vi "Double FFT Mesurament (Control - Init Wave&Window - Snapshot - DoubleFFT - Latency - Low Freq) RT Test.vi"() -> ()   [LabVIEW 2014]
uses:
  <vilib>/Platform/TimedLoop/XDataNode/timing_clust.ctl
  <vilib>/Platform/TimedLoop/XDataNode/nitl_modes.ctl
  <vilib>/Platform/TimedLoop/XDataNode/wakeup.ctl
  <vilib>/FPGAPlugInAG/sbRIO-9636/niLvFpga_Open_sbRIO-9636.vi
  <vilib>/rvi/interface/common/dynamic/niFpgaDynamicAddResources.vi
  <vilib>/Utility/error.llb/Error Cluster From Error Code.vi
  <vilib>/rvi/errors/niLvFpgaAdjustHostInterfaceError.vi
  <vilib>/rvi/interface/common/niFpgaWaitOnOcc.vi
  <vilib>/FPGAPlugInAG/Dynamic/niLvFpga_Run_Dynamic.vi
  <vilib>/FPGAPlugInAG/Dynamic/niLvFpga_Abort_Dynamic.vi
  <vilib>/FPGAPlugInAG/Dynamic/niLvFpga_Reset_Dynamic.vi
  <vilib>/FPGAPlugInAG/Dynamic/niLvFpga_Close_Dynamic.vi
  <vilib>/rvi/interface/nirviOpenFPGA/nirviOpenFPGA.xnode
  FPGA Bitfiles/LaserDistanceSen_FPGATarget_DoubleFFTMesuram_744PzgZsl5A.lvbitx
  FPGA Target/Test VIs/Double FFT Mesurament (Control - Init Wave&Window - Snapshot - DoubleFFT - Latency - Low Freq) test.vi
  <vilib>/rvi/interface/nirviReadWriteControl/nirviReadWriteControl.xnode
  <vilib>/rvi/interface/nirviMethod/nirviMethod.xnode
  <vilib>/Platform/TimedLoop/XDataNode/XDataNode.xnode
  <vilib>/rvi/interface/nirviCloseFPGA/nirviCloseFPGA.xnode
  <vilib>/FPGAPlugInAG/Dynamic/niLvFpga_ConfigureFifo_Dynamic.vi
  <vilib>/rvi/errors/niLvFpgaMergeErrorWithErrorCode.vi
  <vilib>/FPGAPlugInAG/Dynamic/niLvFpga_StartFifo_Dynamic.vi
  <vilib>/rvi/interface/Simulation/niFpgaSimulationCallBeginRW.vi
  <vilib>/FPGAPlugInAG/Dynamic/niLvFpga_ReadFifo_Dynamic.vi
  <vilib>/Platform/TimedLoop/XDataNode/XDNodeRunTimeDep.lvlib
  NiFpgaLv.dll
panel:
  in  "stop":bool
  out "maxbin_secondFFT":i32
  out "maxbin_firstFFT":i32
  out "F_rise":dbl
  out "f_fall":dbl
  out "f_mean":dbl
  out "Velocity (m/s)":dbl
  out "Distance (m)":dbl
  in  "Initial Latency points":u32(slide)=10 scale=0.0..1249.0
  out "Second FFT (bin)":dbl[](graph)
  out "Second Signal (points) - Rising Triangular":dbl[](graph)
  out "Elements Remaining FFT":u32
  out "Elements Remaining Signal":u32
  out "First FFT (bin)":dbl[](graph)
  out "First Signal (points) - Falling Triangular":dbl[](graph)
  in  "Snapshot":bool
  in  "Windowing":T1(ring)
  in  "first bin":i32=15
  in  "last bin":i32=255
  in  "lower limit 2":u32(slide)=725 scale=625.0..738.0
  in  "lower limit 1":u32(slide)=100 scale=0.0..113.0
  # "WARNING:\nOnce pressed wait untill the end of operation"
  # "OFFLINE parameters"
  # "Max Detection FFT bin range"
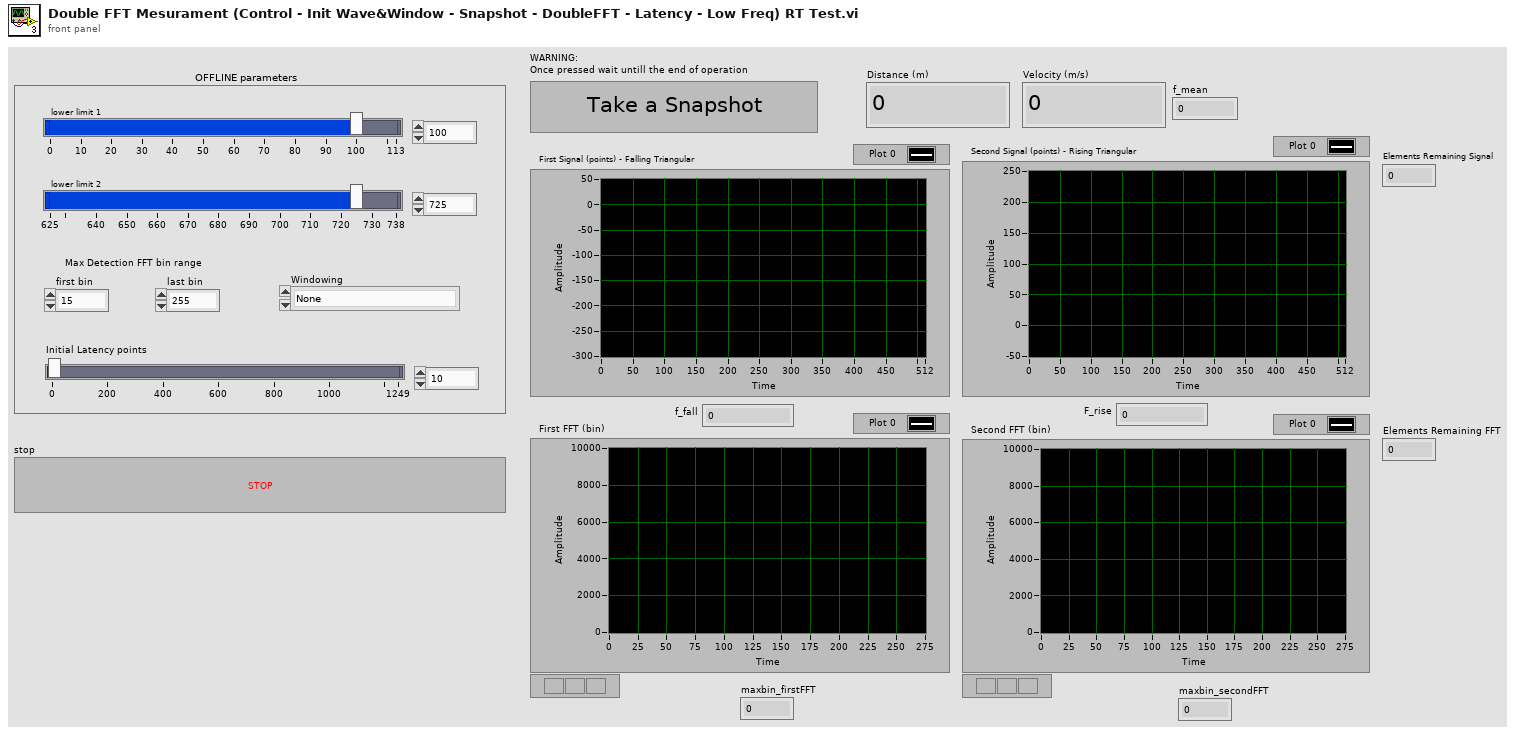
[diagram p1: front panel]
types:
  T1 = enum16{"None", "Hanning", "Hamming", "Blackman", "Blackman-Harris"}
  T2 = typedef "XDNodeRunTimeDep.lvlib/timing_clust.ctl" = cluster{"Expected End [f-1]":u64, "Actual End [f-1]":u64, "Finished Late? [f-1]":bool, "Expected End [i-1]":u64, "Actual End [i-1]":u64, "Finished Late? [i-1]":bool, "Expected Start [i]":u64, "Actual Start [i]":u64, "Expected Start [f]":u64, "Actual Start [f]":u64, "Source Name":string, "Structure Name":string, "Period":i64, "Deadline":i64, "Offset":i64, "Start":i64, "Priority":i32, "Timeout":i32, "Mode":T3, "Wakeup Reason":T4, "Error":errorcluster, "Source Type":string, "Secondary Source Type":string, "Global End Time":u64, "Global Start Time":u64, "Frame Duration":u64, "Iteration Duration":u64, "Assigned CPU":i32, "I/O Scan Engine Mode":u32}
  T3 = typedef "XDNodeRunTimeDep.lvlib/nitl_modes.ctl" = enum32{"No Change", "Process missed periods, maintain original phase", "Discard missed periods, maintain original phase", "Process missed periods, ignore original phase", "Discard missed periods, ignore original phase"}
  T4 = typedef "XDNodeRunTimeDep.lvlib/wakeup.ctl" = enum32{"Normal", "Aborted", "Asynchronous wakeup", "Timing source error", "Timed loop error", "Timeout"}
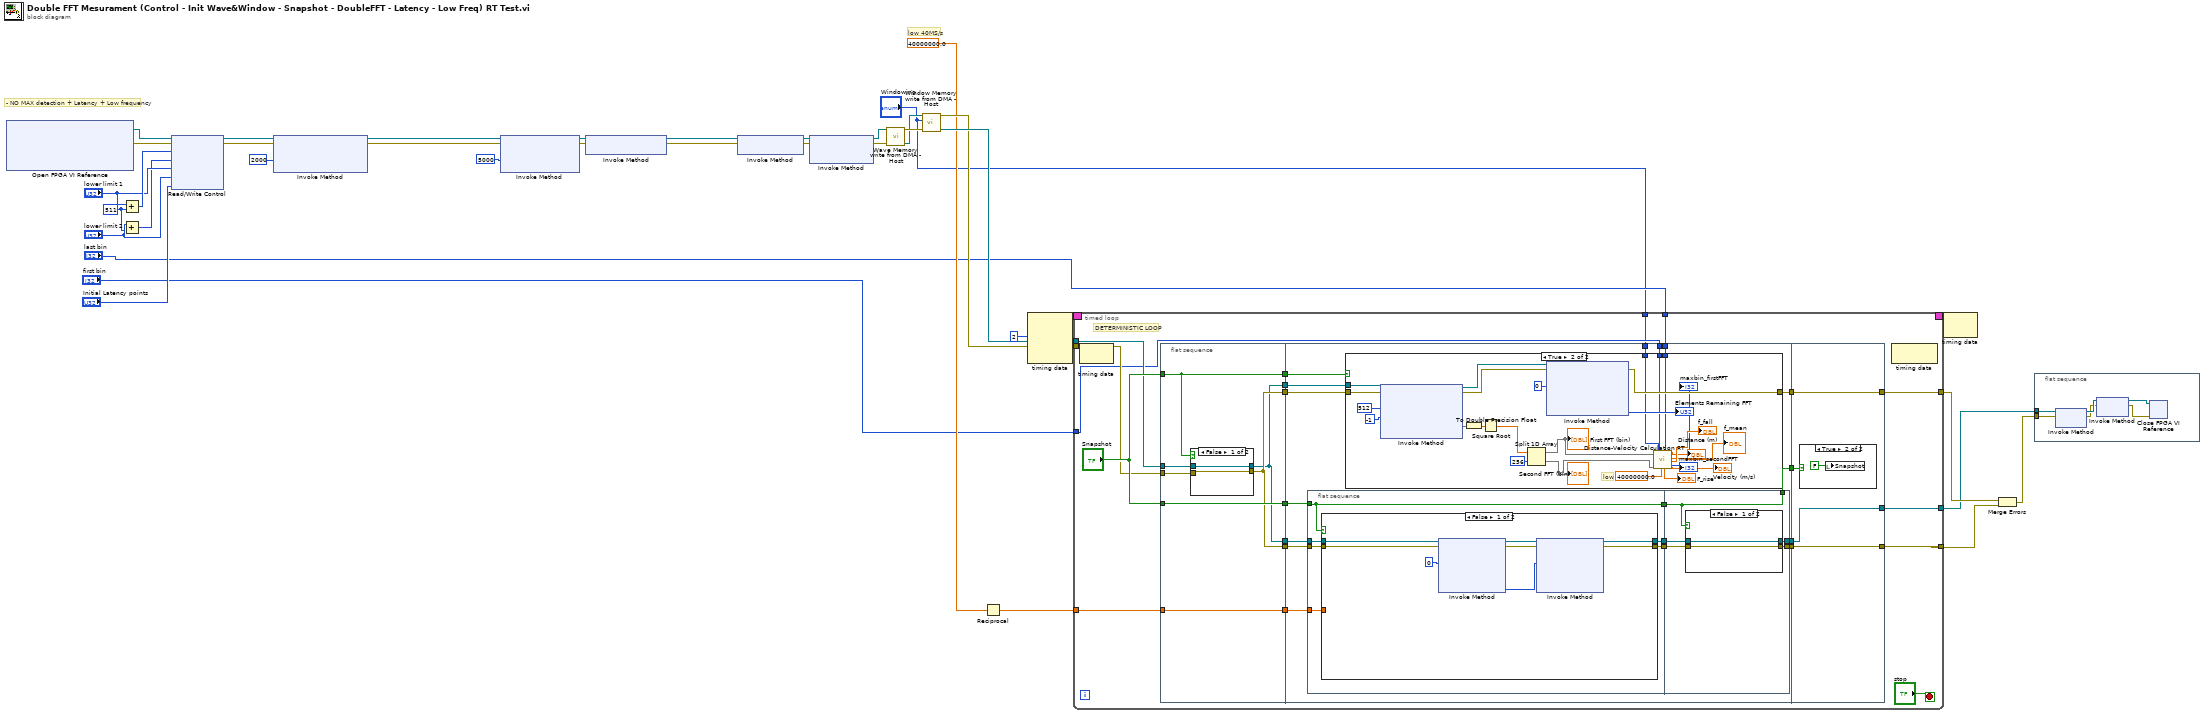
[diagram p0: block diagram]
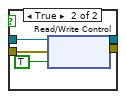
[diagram p2: hidden frame]
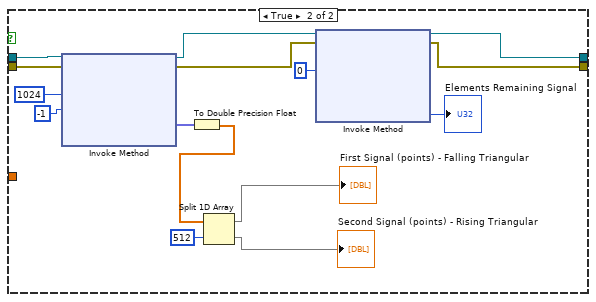
[diagram p3: hidden frame]
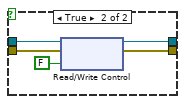
[diagram p4: hidden frame]
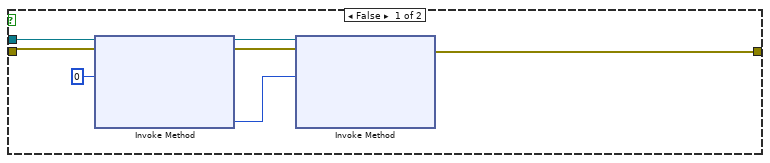
[diagram p5: hidden frame]
diagram:
  w34 = u32 511 ("y")
  # "- NO MAX detection + Latency + Low frequency"
  # "low 40MS/s"
  n1 = xnode "Open FPGA VI Reference"() -> ("FPGA VI Reference Out"=w33:refnum<k20>, "error out"=w32:errorcluster)  [unwired: 2 in]
  n2 = Add(x="lower limit 1", y=w34) -> (x+y=w38:u32)
  n3 = Add(x="lower limit 2", y=w34) -> (x+y=w36:u32)
  n4 = xnode "Read/Write Control"("FPGA VI Reference In"=w33, "error in"=w32, "upper limit 1"=w38, "upper limit 2"=w36, "lower limit 1"="lower limit 1", "lower limit 2"="lower limit 2", "Latency points"="Initial Latency points") -> ("FPGA VI Reference Out"=w29:refnum<k20>, "error out"=w28:errorcluster)
  n5 = xnode "Invoke Method"("FPGA VI Reference In"=w29, "error in"=w28, "Requested Depth"=u32 2000) -> ("FPGA VI Reference Out"=w4:refnum<k20>, "error out"=w5:errorcluster)  [unwired: 1 out]
  n6 = xnode "Invoke Method"("FPGA VI Reference In"=w4, "error in"=w5, "Requested Depth"=u32 5000) -> ("FPGA VI Reference Out"=w18:refnum<k20>, "error out"=w19:errorcluster)  [unwired: 1 out]
  n7 = xnode "Invoke Method"("FPGA VI Reference In"=w18, "error in"=w19) -> ("FPGA VI Reference Out"=w2:refnum<k20>, "error out"=w3:errorcluster)
  n8 = xnode "Invoke Method"("FPGA VI Reference In"=w2, "error in"=w3) -> ("FPGA VI Reference Out"=w16:refnum<k20>, "error out"=w17:errorcluster)
  n9 = xnode "Invoke Method"("FPGA VI Reference In"=w16, "error in"=w17) -> ("FPGA VI Reference Out"=w22:refnum<k20>, "error out"=w21:errorcluster)  [unwired: 1 in]
  n10 = call "Wave Memory write from DMA - Host.vi"("error in"=w21, "FPGA VI Reference In"=w22) -> ("FPGA VI Reference Out"=w7:refnum<k20>, "error out"=w20:errorcluster)  [unwired: 7 in, 1 out]
  n11 = call "Window Memory write from DMA - Host.vi"("error in"=w20, "Enum"="Windowing", "FPGA VI Reference In"=w7) -> ("FPGA VI Reference Out"=w31:refnum<k20>, "error out"=w30:errorcluster)  [unwired: 5 in, 2 out]
  n12 = Reciprocal(x=40000000.0 ("Sample Rate (S/s)")) -> (1/x=w24:dbl)
  n13 = node-c288(i64 2 ("Period")) -> (w15:T2)  [unwired: 3 in]
  n14 = timed-loop {
    tunnel: w31 -> [w55]
    tunnel: w30 -> [w56]
    tunnel: [w58] -> w12
    tunnel: w24 -> [w60]
    tunnel: [w59] -> w11
    timing: w15 -> [_]
    timing-out: [_] -> w14
    tunnel: "first bin" -> [w44]
    tunnel: "last bin" -> [w43]
    tunnel: [w41] -> w6
    tunnel: "Windowing" -> [w39]
    stop <- "stop" stop-if-true
    # "DETERMINISTIC LOOP"
    n15 = node-c288() -> ()  [unwired: 1 in, 1 out]
    n16 = flat-sequence {
      tunnel: w55 -> [w65]
      tunnel: w56 -> [w66]
      tunnel: "Snapshot" -> [w63]
      tunnel: "Snapshot" -> [w68]
      tunnel: w60 -> [w69]
      tunnel: [w67] -> w54
      tunnel: [w69] -> w53
      tunnel: [w68] -> w52
      tunnel: [w63] -> w51
      tunnel: [w67] -> w50
      tunnel: [w64] -> w49
      tunnel: [w64] -> w48
      tunnel: w54 -> [w89]
      tunnel: w53 -> [w88]
      tunnel: w52 -> [w82]
      tunnel: w51 -> [w85]
      tunnel: w50 -> [w84]
      tunnel: w49 -> [w83]
      tunnel: w48 -> [w90]
      tunnel: [w87] -> w47
      tunnel: [w86] -> w46
      tunnel: [w81] -> w45
      tunnel: w44 -> [w80]
      tunnel: w43 -> [w79]
      tunnel: [w78] -> w40
      tunnel: w39 -> [w77]
      tunnel: [w170] -> w58
      tunnel: [w171] -> w59
      tunnel: w47 -> [w171]
      tunnel: w46 -> [w170]
      tunnel: w45 -> [w169]
      tunnel: [w168] -> w41
      tunnel: w40 -> [w168]
      frame #0 {
        n17 = case shown="False" w63 {
          tunnel: [w70 w75] -> w67
          tunnel: w66 -> [w70 w74]
          tunnel: w65 -> [w71 w73]
          tunnel: [w71 w72] -> w64
          frame False {
          }
          frame True {
            n18 = xnode "Read/Write Control"("FPGA VI Reference In"=w73, "error in"=w74, "snapshot"=TRUE) -> ("FPGA VI Reference Out"=w72:refnum<k20>, "error out"=w75:errorcluster)
          }
        }
      }
      frame #1 {
        n19 = flat-sequence {
          tunnel: w90 -> [w99]
          tunnel: w89 -> [w98]
          tunnel: w88 -> [w97]
          tunnel: w82 -> [w94]
          tunnel: [w96] -> w93
          tunnel: [w95] -> w92
          tunnel: [w94] -> w91
          tunnel: [w125] -> w86
          tunnel: w93 -> [w127]
          tunnel: w92 -> [w126]
          tunnel: w91 -> [w124]
          tunnel: [w124] -> w81
          tunnel: [w123] -> w78
          frame #0 {
            n20 = case shown="False" w94 {
              tunnel: w99 -> [w106 w122]
              tunnel: w98 -> [w104 w121]
              tunnel: [w103 w114] -> w95
              tunnel: w97 -> [_ _]
              tunnel: [w100 w113] -> w96
              frame False {
                n21 = xnode "Invoke Method"("FPGA VI Reference In"=w106, "error in"=w104, "Number of Elements"=u32 0) -> ("FPGA VI Reference Out"=w102:refnum<k20>, "error out"=w101:errorcluster, "Elements Remaining"=w105:u32)  [unwired: 1 in, 1 out]
                n22 = xnode "Invoke Method"("FPGA VI Reference In"=w102, "error in"=w101, "Number of Elements"=w105) -> ("FPGA VI Reference Out"=w100:refnum<k20>, "error out"=w103:errorcluster)  [unwired: 1 in, 2 out]
              }
              frame True {
                n23 = xnode "Invoke Method"("FPGA VI Reference In"=w122, "error in"=w121, "Number of Elements"=u32 1024, "Timeout (ms)"=-1) -> ("FPGA VI Reference Out"=w116:refnum<k20>, "error out"=w115:errorcluster, "Data"=w118:fxp<+/-,12,12>[])  [unwired: 1 out]
                n24 = To Double Precision Float(number=w118) -> (double precision float=w111:dbl[])
                n25 = Split 1D Array(array=w111, index=512) -> (first subarray=→"First Signal (points) - Falling Triangular":dbl[], second subarray=→"Second Signal (points) - Rising Triangular":dbl[])
                n26 = xnode "Invoke Method"("FPGA VI Reference In"=w116, "error in"=w115, "Number of Elements"=u32 0) -> ("FPGA VI Reference Out"=w113:refnum<k20>, "error out"=w114:errorcluster, "Elements Remaining"=→"Elements Remaining Signal":u32)  [unwired: 1 in, 1 out]
              }
            }
          }
          frame #1 {
            n27 = case shown="False" w124 {
              tunnel: [w129 w132] -> w125
              tunnel: w127 -> [w128 w133]
              tunnel: w126 -> [w129 w131]
              tunnel: [w128 w130] -> w123
              frame False {
              }
              frame True {
                n28 = xnode "Read/Write Control"("FPGA VI Reference In"=w133, "error in"=w131, "snapshot"=FALSE) -> ("FPGA VI Reference Out"=w130:refnum<k20>, "error out"=w132:errorcluster)
              }
            }
          }
        }
        n29 = case shown="True" w85 {
          tunnel: w83 -> [w140 w162]
          tunnel: w84 -> [w137 w163]
          tunnel: [w136 w161] -> w87
          tunnel: w80 -> [_ w145]
          tunnel: w79 -> [_ w146]
          tunnel: w77 -> [_ w142]
          frame False {
            n30 = xnode "Invoke Method"("FPGA VI Reference In"=w140, "error in"=w137, "Number of Elements"=u32 0) -> ("FPGA VI Reference Out"=w138:refnum<k20>, "error out"=w135:errorcluster, "Elements Remaining"=w139:u32)  [unwired: 1 in, 1 out]
            n31 = xnode "Invoke Method"("FPGA VI Reference In"=w138, "error in"=w135, "Number of Elements"=w139) -> ("error out"=w136:errorcluster)  [unwired: 1 in, 3 out]
          }
          frame True {
            # "low"
            n32 = xnode "Invoke Method"("FPGA VI Reference In"=w162, "error in"=w163, "Number of Elements"=u32 512, "Timeout (ms)"=-1) -> ("FPGA VI Reference Out"=w159:refnum<k20>, "error out"=w160:errorcluster, "Data"=w165:fxp<+,44,44>[])  [unwired: 1 out]
            n33 = To Double Precision Float(number=w165) -> (double precision float=w164:dbl[])
            n34 = Square Root(x=w164) -> (sqrt(x)=w156:dbl[])
            n35 = Split 1D Array(array=w156, index=256) -> (first subarray=w154:dbl[], second subarray=w153:dbl[])
            "First FFT (bin)" <- w154
            "Second FFT (bin)" <- w153
            n36 = xnode "Invoke Method"("FPGA VI Reference In"=w159, "error in"=w160, "Number of Elements"=u32 0) -> ("error out"=w161:errorcluster, "Elements Remaining"=→"Elements Remaining FFT":u32)  [unwired: 1 in, 2 out]
            n37 = call "Distance-Velocity Calculation RT.vi"("First FFT"=w154, "Second FFT"=w153, "Windowing"=w142, "first FFT bin"=w145, "Sample Rate (S/s)"=40000000.0, "last FFT bin"=w146) -> ("F_rise"=→"F_rise":dbl, "maxbin_firstFFT"=→"maxbin_firstFFT":i32, "maxbin_secondFFT"=→"maxbin_secondFFT":i32, "Distance (m)"=→"Distance (m)":dbl, "f_mean"=→"f_mean":dbl, "F_fall"=→"f_fall":dbl, "Velocity (m/s)"=→"Velocity (m/s)":dbl)  [unwired: 7 in]
          }
        }
      }
      frame #2 {
        n38 = case shown="True" w169 {
          frame False {
          }
          frame True {
            n39 = local write "Snapshot"(FALSE ("Snapshot")) -> ()
          }
        }
      }
    }
    n40 = node-c288() -> ()  [unwired: 1 in, 1 out]
  }
  n41 = node-c288(w14) -> ()  [unwired: 1 out]
  n42 = Merge Errors(w11, w12) -> (w25:errorcluster)
  n43 = flat-sequence {
    tunnel: w25 -> [w178]
    tunnel: w6 -> [w173]
    frame #0 {
      n44 = xnode "Invoke Method"("FPGA VI Reference In"=w173, "error in"=w178) -> ("FPGA VI Reference Out"=w175:refnum<k20>, "error out"=w174:errorcluster)
      n45 = xnode "Invoke Method"("FPGA VI Reference In"=w175, "error in"=w174) -> ("FPGA VI Reference Out"=w176:refnum<k20>, "error out"=w177:errorcluster)
      n46 = xnode "Close FPGA VI Reference"("FPGA VI Reference In"=w176, "error in"=w177) -> ()  [unwired: 1 out]
    }
  }
